vi "Draw Element.vi"(8 "Error In":errorcluster, 10 "Element To Display":T1[](array[typedef]), 11 "Frame In":u32[][](array[numeric])) -> (0 "Error Out":errorcluster, 2 "Frame Changed?":bool, 3 "Frame Out":u32[][](array[numeric]))   [LabVIEW 2021, in "Display Manager.lvclass"]
uses:
  Display Manager.lvclass
  Display Element/Public/Controls/Pixel.ctl
  Display Utilities/Public/Controls/2D Coordinates.ctl
  Display Manager.lvclass/Display Manager.ctl
  Display Utilities/Display Utilities.lvlib
  Display Element/Display Element.lvclass
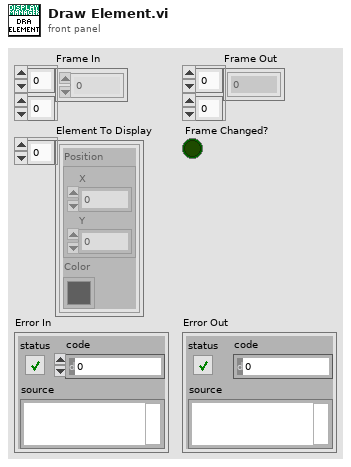
[diagram p1: front panel]
types:
  T1 = typedef "Display Element.lvclass/Pixel.ctl" = cluster{"Position":T2, "Color":u32}
  T2 = typedef "Display Utilities.lvlib/2D Coordinates.ctl" = cluster{"X":i32, "Y":i32}
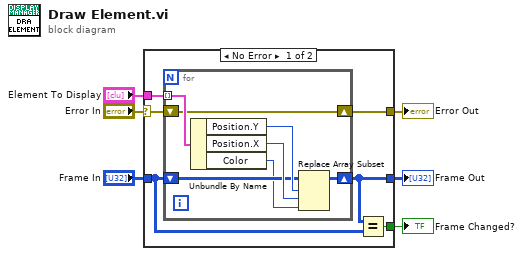
[diagram p0: block diagram]
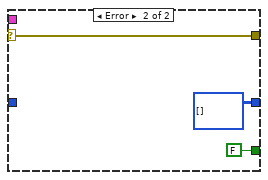
[diagram p2: hidden frame]
diagram:
  n1 = case shown="No Error" "Error In" {
    selector: "Error In" -> [w11 w22]
    tunnel: [w12 w22] -> w6
    tunnel: "Frame In" -> [w8 _]
    tunnel: [w9 u32[][] [] ("Frame In")] -> w4
    tunnel: "Element To Display" -> [w10 _]
    tunnel: [w7 FALSE] -> w1
    frame No Error {
      n2 = for {
        tunnel: w10 -> [w19] mode=indexing
        shift-right: [w17] -> w9
        shift-left: w8 -> [w14]
        shift-right: [w18] -> w12
        shift-left: w11 -> [w18]
        n3 = Unbundle By Name(w19) -> ("Position.Y"=w16:i32, "Position.X"=w15:i32, "Color"=w13:u32)
        n4 = Replace Array Subset(array=w14, new element=w13, index (row)=w16, index (col)=w15) -> (w17:u32[][])
      }
      n5 = Equal?(x=w9, y=w8) -> (x = y?=w7:bool)
    }
    frame Error {
    }
  }
  "Error Out" <- w6
  "Frame Out" <- w4
  "Frame Changed?" <- w1
